vi "LSX Get Sm Hdi Button.vi"(7 "lMaxLen":i32, 8 "error in (no error)":errorcluster, 9 "pcFunction":string, 10 "lButtonNr":i32, 11 "lLSID":i32) -> (0 "error out":errorcluster, 1 "pcFunction out":string, 3 "function return":i32)   [LabVIEW 2018, in "Tango.lvlib"]
doc: "TANGOAPI int TANGOCALL LSX_GetSmHdiButton (int lLSID, int lButtonNr, char *pcFunction, int lMaxLen);"
uses:
  <userlib>/Tango/Tango.lvlib
  <userlib>/Tango/Tango_DLL.dll
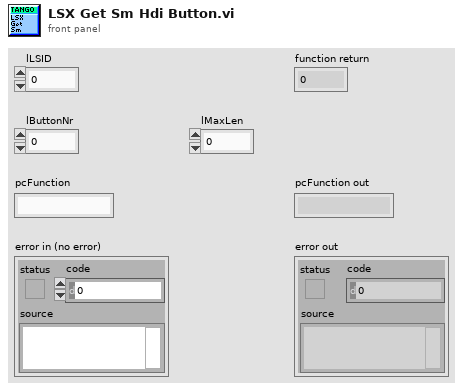
[diagram p1: front panel]
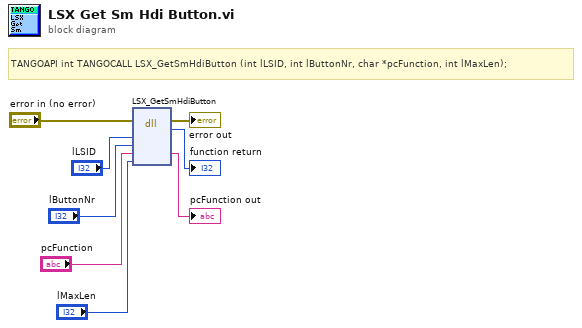
[diagram p0: block diagram]
diagram:
  # "TANGOAPI int TANGOCALL LSX_GetSmHdiButton (int lLSID, int lButtonNr, char *pcFunction, int lMaxLen);"
  n1 = dll-call lib="C:/Program Files (x86)/National Instruments/LabVIEW 2018/user.lib/Tango/Tango_DLL.*" fn="LSX_GetSmHdiButton"(error in="error in (no error)", "lLSID"="lLSID", "lButtonNr"="lButtonNr", "pcFunction"="pcFunction", "lMaxLen"="lMaxLen") -> (error out=→"error out":errorcluster, →"function return":i32, "pcFunction"=→"pcFunction out":string)  [unwired: 5 in, 1 out]
